vi "Unitary_Test_Set.vi"() -> (0 "Test_passed":bool)   [LabVIEW 2015]
panel:
  in  "bad values":string[](array[string])=["0", "hola", "0,000000", "false", "0,000000"]
  in  "bad variables":string[](array[string])=["FAKEVAR", "stringout", "time", "booleanout", "doubleout"]
  out "hidden":errorcluster
  out "returned values":string[](array[string])=["-47", "\"adios\"", "true", "0.100000"]
  in  "values to set":string[](array[string])=["-47", "adios", "true", "0.1"]
  in  "Expected values":string[](array[string])=["-47", "\"adios\"", "true", "0.100000"]
  out "error 2 must FAIL":errorcluster={"status"=TRUE, "code"=1, "source"="Invoke Node in set.vi->Unitary_Test_Set.vi\n<APPEND>\nMethod Name: <b>Control Value:Get</b>\n\n\"FAKEVAR\" not found\nwhile reading variable: FAKEVAR\nOn expid:TestOK"}
  in  "variables":string[](array[string])=["intin", "stringin", "booleanin", "doublein"]
  out "error 1 must be OK":errorcluster
  out "hidden3":errorcluster
  out "hidden":errorcluster
  in  "Experience ID1":string="TestOK"
  out "Test_OK":bool[](array[boolean])=[FALSE, TRUE]
  # "Test basic methods with some testing plant"
  # "test 1 multiple reads OK"
  # "test 2 wrogn variables"
  # "test 3 multiple formats of double"
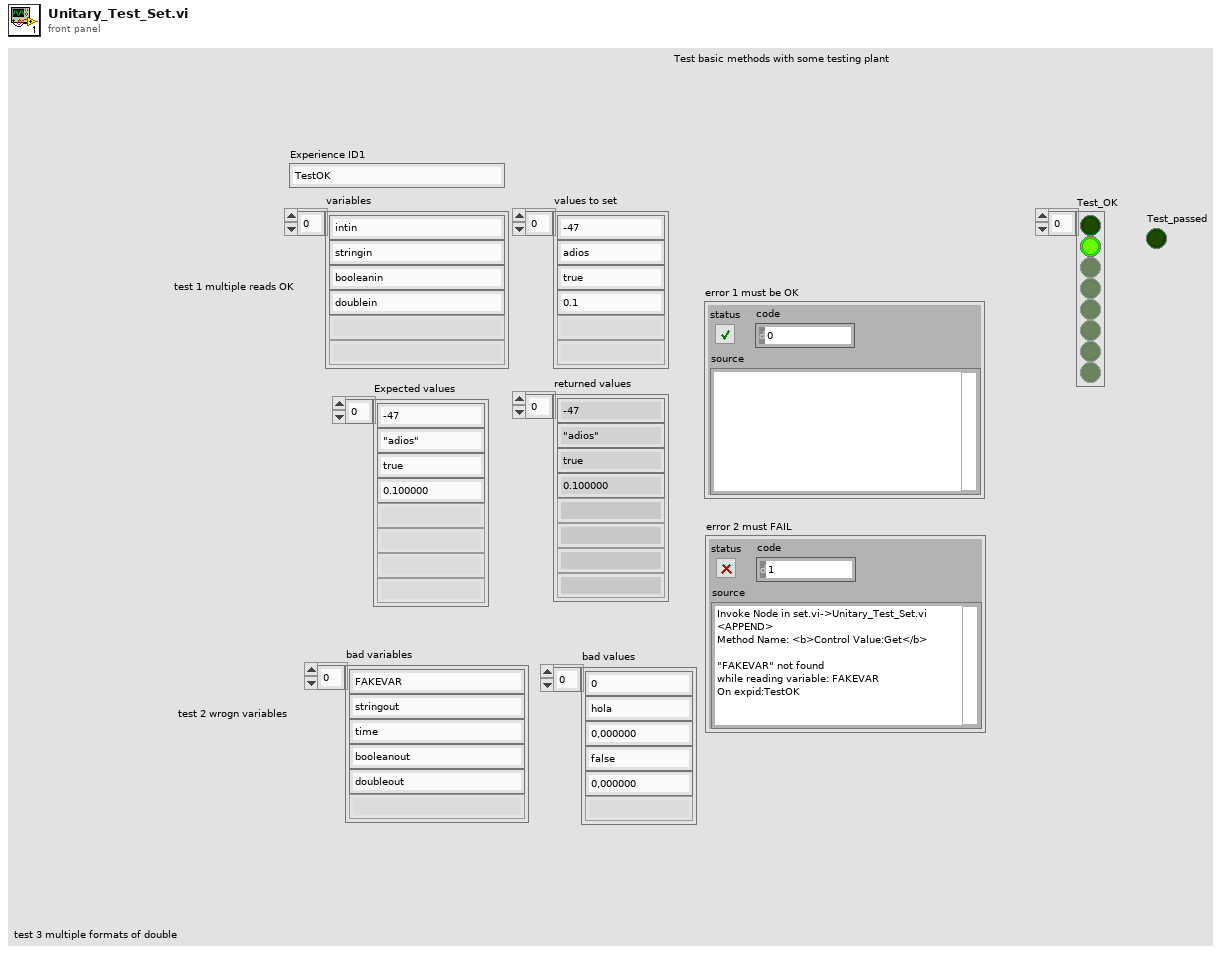
[diagram p1: front panel]
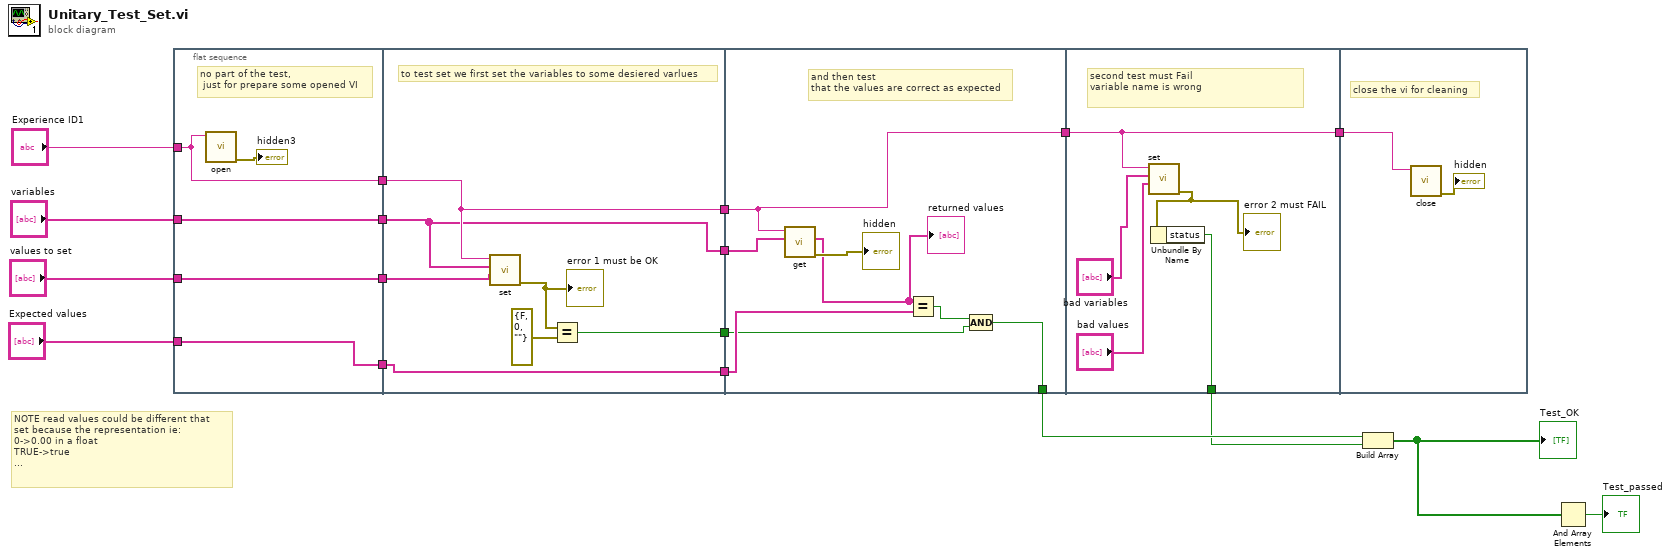
[diagram p0: block diagram]
diagram:
  # "NOTE read values could be different that \nset because the representation ie:\n0->0.00 in a float\nTRUE->true\n..."
  n1 = flat-sequence {
    tunnel: "Experience ID1" -> [w22]
    tunnel: [w22] -> w5
    tunnel: [w21] -> w4
    tunnel: "variables" -> [w21]
    tunnel: [w20] -> w3
    tunnel: "Expected values" -> [w20]
    tunnel: [w19] -> w2
    tunnel: "values to set" -> [w19]
    tunnel: w5 -> [w25]
    tunnel: w4 -> [w24]
    tunnel: w3 -> [w27]
    tunnel: w2 -> [w28]
    tunnel: [w27] -> w11
    tunnel: [w26] -> w10
    tunnel: [w25] -> w9
    tunnel: [w24] -> w8
    tunnel: [w31] -> w12
    tunnel: w11 -> [w36]
    tunnel: w10 -> [w34]
    tunnel: w9 -> [w31]
    tunnel: w8 -> [w38]
    tunnel: [w33] -> w7
    tunnel: w12 -> [w42]
    tunnel: [w42] -> w15
    tunnel: [w43] -> w6
    tunnel: w15 -> [w44]
    frame #0 {
      # "no part of the test,\n just for prepare some opened VI"
      n2 = call "open.vi"("Experience ID"=w22) -> ("error out"=→"hidden3":errorcluster)  [unwired: 8 in, 2 out]
    }
    frame #1 {
      # "to test set we first set the variables to some desiered varlues"
      n3 = call "set.vi"("values"=w28, "variables"=w24, "Experience ID"=w25) -> ("error out"=w29:errorcluster)  [unwired: 8 in]
      "error 1 must be OK" <- w29
      n4 = Equal?(x=w29, y=errorcluster {"status"=FALSE, "code"=0, "source"=""} ("error out")) -> (x = y?=w26:bool)
    }
    frame #2 {
      # "and then test\nthat the values are correct as expected"
      n5 = call "get.vi"("variables"=w38, "Experience ID"=w31) -> ("error out"=→"hidden":errorcluster, "values"=w32:string[])  [unwired: 7 in, 1 out]
      "returned values" <- w32
      n6 = Equal?(x=w32, y=w36) -> (x = y?=w35:bool)
      n7 = Compound Arithmetic op=AND(w35, w34) -> (w33:bool)
    }
    frame #3 {
      # "second test must Fail\nvariable name is wrong"
      n8 = call "set.vi"("values"="bad values", "variables"="bad variables", "Experience ID"=w42) -> ("error out"=w39:errorcluster)  [unwired: 8 in]
      "error 2 must FAIL" <- w39
      n9 = Unbundle By Name(w39) -> ("status"=w43:bool)
    }
    frame #4 {
      # "close the vi for cleaning"
      n10 = call "close.vi"("Experience ID"=w44) -> ("error out"=→"hidden":errorcluster)  [unwired: 10 in]
    }
  }
  n11 = Build Array(w7, w6) -> (w17:bool[])
  "Test_OK" <- w17
  n12 = And Array Elements(Boolean array=w17) -> (logical AND=→"Test_passed":bool)
